vi "TWM Client Cmd Define QPMX.vi"(1 "Switch mode":T1(ring), 2 "Trigger polarity":enum16{"Positive", "Negative", "No change"}(ring)=enum."No change", 4 "Timing delays":i64[](array[numeric]), 5 "timeout [ms]":i32=5000, 6 "Sequence":bool[][](array[boolean]), 7 "end of packet key":string="TWM:command:EndOfPacket", 8 "error in":errorcluster, 9 "Internal timer (s)":dbl=nan, 10 "Short circuit delay (s)":dbl=nan, 11 "handle":i32) -> (0 "error out":errorcluster, 3 "handle out":i32)   [LabVIEW 2020, in "TWM Client.lvlib"]
doc: "This will define QPMX multiplexer sequence and properties. It's equivalent to manual setup of QPMX in multiplexer panel. If some inputs are not wired, particular values are not changed."
uses:
  TWM Client.lvlib
  octave/infolib/String.vi
  octave/infolib/EXT.vi
  octave/infolib/2D I64.vi
  octave/infolib/1D I64.vi
  octave/infolib/infolib.lvlib
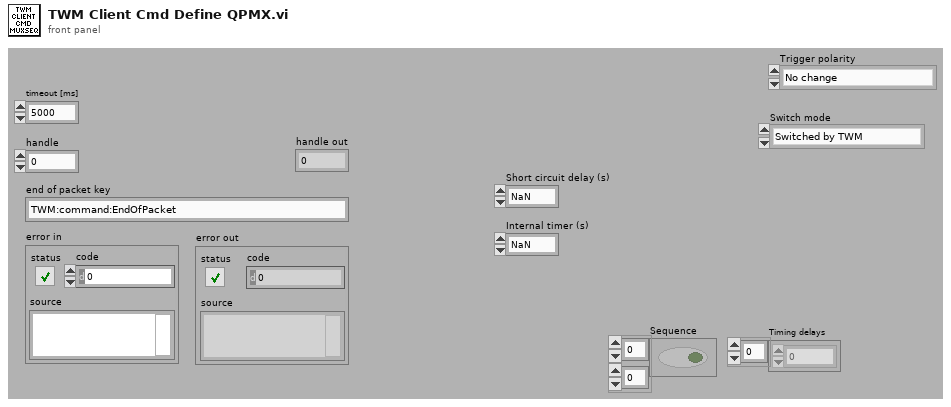
[diagram p1: front panel]
types:
  T1 = enum16{"Switched by TWM", "Switched by internal clock", "Switched by external clock", "No change"}
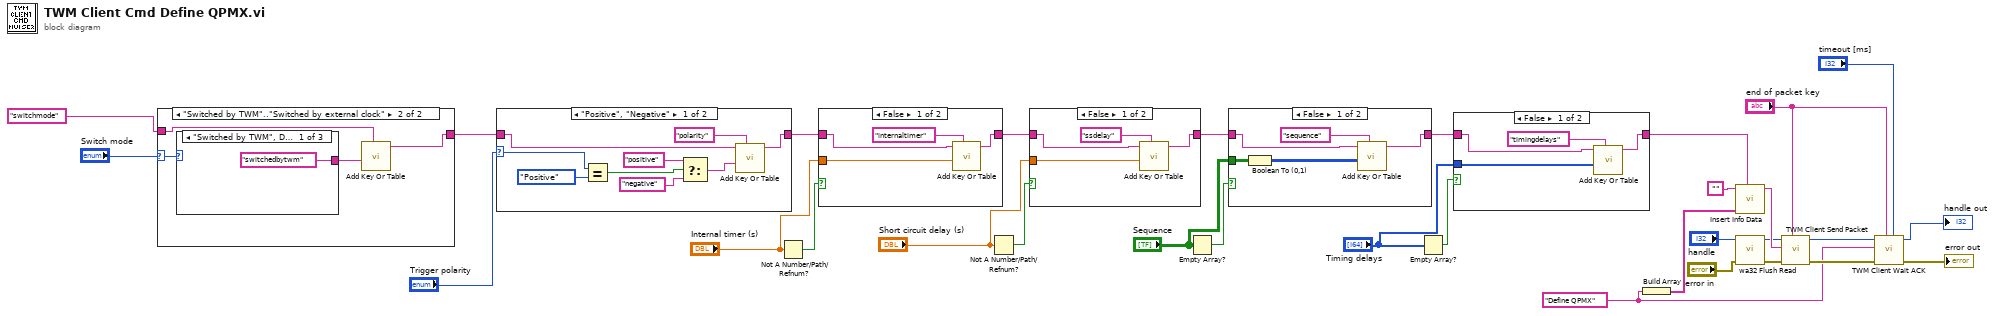
[diagram p0: block diagram]
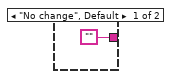
[diagram p6: hidden frame]
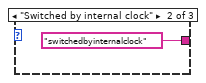
[diagram p7: hidden frame]
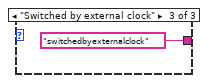
[diagram p8: hidden frame]
diagram:
  w24 = "Define QPMX" ("section name")
  n1 = case shown="\"Switched by TWM\"..\"Switched by external clock\"" "Switch mode" {
    selector: "Switch mode" -> [_ w33]
    tunnel: "switchmode" ("key description") -> [_ w35]
    tunnel: ["" w34] -> w14
    frame "No change", Default {
    }
    frame "Switched by TWM".."Switched by external clock" {
      n2 = case shown="\"Switched by TWM\", Default" w33 {
        tunnel: ["switchedbytwm" ("key description") "switchedbyinternalclock" ("key description") "switchedbyexternalclock" ("key description")] -> w36
        frame "Switched by TWM", Default {
        }
        frame "Switched by internal clock" {
        }
        frame "Switched by external clock" {
        }
      }
      n3 = call-poly "Add Key Or Table.vi"("key description"=w35, "string"=w36) -> ("info data out"=w34:string)  [unwired: 8 in, 1 out]
    }
  }
  n4 = case shown="\"Positive\", \"Negative\"" "Trigger polarity" {
    selector: "Trigger polarity" -> [w43 _]
    tunnel: w14 -> [w41 w49]
    tunnel: [w40 w49] -> w13
    frame "Positive", "Negative" {
      n5 = Equal?(x=w43, y=enum16{"Positive", "Negative", "No change"}."Positive" ("Trigger polarity")) -> (x = y?=w44:bool)
      n6 = Select(t="positive" ("key description"), s=w44, f="negative" ("key description")) -> (s? t:f=w42:string)
      n7 = call-poly "Add Key Or Table.vi"("key description"="polarity", "string"=w42, "info data"=w41) -> ("info data out"=w40:string)  [unwired: 7 in, 1 out]
    }
    frame "No change", Default {
    }
  }
  n8 = Not A Number/Path/Refnum?(number/path/refnum="Internal timer (s)") -> (NaN/Path/Refnum?=w7:bool)
  n9 = case shown="False" w7 {
    tunnel: w13 -> [w52 w54]
    tunnel: [w51 w54] -> w12
    tunnel: "Internal timer (s)" -> [w50 _]
    frame False {
      n10 = call-poly "Add Key Or Table.vi"("key description"="internaltimer", "numeric"=w50, "info data"=w52) -> ("info data out"=w51:string)  [unwired: 7 in, 1 out]
    }
    frame True {
    }
  }
  n11 = Not A Number/Path/Refnum?(number/path/refnum="Short circuit delay (s)") -> (NaN/Path/Refnum?=w5:bool)
  n12 = case shown="False" w5 {
    tunnel: w12 -> [w57 w59]
    tunnel: [w56 w59] -> w11
    tunnel: "Short circuit delay (s)" -> [w55 _]
    frame False {
      n13 = call-poly "Add Key Or Table.vi"("key description"="ssdelay", "numeric"=w55, "info data"=w57) -> ("info data out"=w56:string)  [unwired: 7 in, 1 out]
    }
    frame True {
    }
  }
  n14 = Empty Array?(array="Sequence") -> (empty?=w3:bool)
  n15 = case shown="False" w3 {
    tunnel: "Sequence" -> [w63 _]
    tunnel: w11 -> [w61 w65]
    tunnel: [w60 w65] -> w10
    frame False {
      n16 = Boolean To (0,1)(Boolean=w63) -> (0, 1=w62:i16[][])
      n17 = call-poly "Add Key Or Table.vi"("key description"="sequence", "numeric"=w62, "info data"=w61) -> ("info data out"=w60:string)  [unwired: 8 in]
    }
    frame True {
    }
  }
  n18 = Empty Array?(array="Timing delays") -> (empty?=w2:bool)
  n19 = case shown="False" w2 {
    tunnel: [w69 w70] -> w21
    tunnel: "Timing delays" -> [w67 _]
    tunnel: w10 -> [w66 w70]
    frame False {
      n20 = call-poly "Add Key Or Table.vi"("key description"="timingdelays", "numeric"=w67, "info data"=w66) -> ("info data out"=w69:string)  [unwired: 7 in, 1 out]
    }
    frame True {
    }
  }
  n21 = Build Array(w24) -> (w30:string[])
  n22 = call "Insert Info Data.vi"("info data to insert"=w21, "sections"=w30, "info data"="") -> ("info data out"=w31:string)  [unwired: 7 in, 1 out]
  n23 = call "wa32 Flush Read.vi"("error in"="error in", "handle"="handle") -> ("error out"=w19:errorcluster, "handle out"=w18:i32)  [unwired: 7 in, 1 out]
  n24 = call "TWM Client Send Packet.vi"("end of packet key"="end of packet key", "error in"=w19, "command string"=w31, "handle"=w18) -> ("error out"=w26:errorcluster, "handle out"=w23:i32)  [unwired: 6 in]
  n25 = call "TWM Client Wait ACK.vi"("timeout [ms] (3000)"="timeout [ms]", "key string"="end of packet key", "error in"=w26, "command header"=w24, "handle"=w23) -> ("error out"=→"error out":errorcluster, "handle out"=→"handle out":i32)  [unwired: 5 in]
